vi "broken add.vi"(10 "y":dbl, 11 "x":dbl) -> (3 "x+y":dbl)   [LabVIEW 2013]
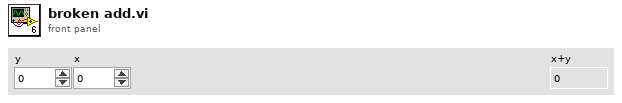
[diagram p1: front panel]
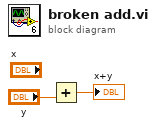
[diagram p0: block diagram]
diagram:
  n1 = Add(y="y") -> (x+y=→"x+y":dbl)  [unwired: 1 in]
